vi "PCert-Container-TellActor.vi"(8 "error in (no error)":errorcluster, 9 "Payload":string, 10 "Command":string, 11 "ERP-Container-UI in":refnum<class "PCert-Container-UI.lvclass">) -> (0 "error out":errorcluster, 3 "ERP-Container-UI out":refnum<class "PCert-Container-UI.lvclass">)   [LabVIEW 2013, in "PCert-Container-UI.lvclass"]
uses:
  PCert-Container-UI.lvclass
  PCert-Container-UI.lvclass/PCert-Container-UI.ctl
  ftw-dataflow/Actor/src/Connector/FTW-ActorConnector.lvclass
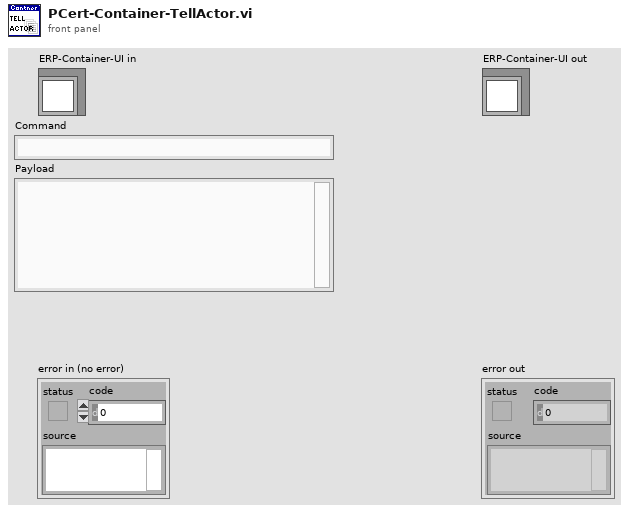
[diagram p1: front panel]
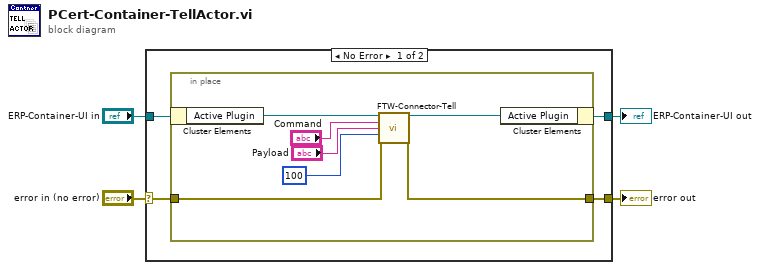
[diagram p0: block diagram]
diagram:
  n1 = case shown="No Error" "error in (no error)" {
    selector: "error in (no error)" -> [w8 w17]
    tunnel: [w7 w17] -> w3
    tunnel: [w5 w16] -> w1
    tunnel: "ERP-Container-UI in" -> [w6 w16]
    frame No Error {
      n2 = in-place {
        in-place-border: w8 -> [w11]
        in-place-border: [w10] -> w7
        n3 = in-place-cluster #1(w6) -> ("Active Plugin"=w15:refnum<class "FTW-ActorConnector.lvclass">)
        n4 = call "FTW-Connector-Tell.vi"("FTW Actor Connector"=w15, "Message Header"="Command", "Message Body"="Payload", "Timeout"=100, "error in"=w11) -> ("FTW Actor Connector out"=w12:refnum<class "FTW-ActorConnector.lvclass">, "error out"=w10:errorcluster)  [unwired: 8 in, 1 out]
        n5 = in-place-cluster #1("Active Plugin"=w12) -> (w5:refnum<class "PCert-Container-UI.lvclass">)
      }
    }
    frame Error {
    }
  }
  "error out" <- w3
  "ERP-Container-UI out" <- w1
